vi "Mindsensors Numeric Pad Config.vi"(10 "Node Data":T1, 11 "NXT":T3) -> ()   [LabVIEW 2010]
uses:
  <vilib>/NXT/Subs/LVHSConnector.ctl
  Datatypes/Node.ctl
  UI Controls/PlugInControls/Pluginbackground.ctl
  <vilib>/NXT/Block Support/nxt.ctl
  <vilib>/NXT/Block Support/HWPage.SensorMode.ctl
  <vilib>/Utility/miscctls.llb/LVPointTypeDef.ctl
  <vilib>/NXT/Block Support/HWPage.SensorType.ctl
  ConvertNodeAddrSensor.vi
panel:
  in  "Node Data 2":T1
  out "error out":errorcluster
  out "NXTObject dup":T2 {"nxtIterHandle" format="%08x"; "modIterHandle" format="%08x"; "moduleHandle" format="%08x"; "fileIterHandle" format="%08x"; "fileHandle" format="%08x"; "nxtHandle" format="%08x"}
  in  "Numeric Pad":string
  out "Input Port":sgl
  out "Device Addr":u8 format="%x"
  out "number":i8
  out "#":bool
  out "9":bool
  out "6":bool
  out "3":bool
  out "0":bool
  out "8":bool
  out "5":bool
  out "2":bool
  out "*":bool
  out "7":bool
  out "4":bool
  out "1":bool
  out "?":dbl format="%#.2g"
  in  "Device Address":string
  in  "NXT Port":string
  in  "Name":string
  out "Headline":string="Type (auto populated)"
  in  "Sensor Parameters":string
  in  "Instance Specific Data":cluster{"Example Data":dbl}
  in  "Reset":bool
  in  "Save":bool
  in  "Stop":bool
  out "Background":T4=TRUE
  # "<- No controls below this line"
  # "Common controls such as Buttons, Rings, Sliders, Graphs, Decorations, etc can be found in the <labview>\\Targets\\NI\\NXT\\NXT Toolkit\\Schematic Editor\\UI Controls\\Plugin Controls\\ folder. Use these controls when possible to ensure a consistent look and feel with LabVIEW Education Edition."
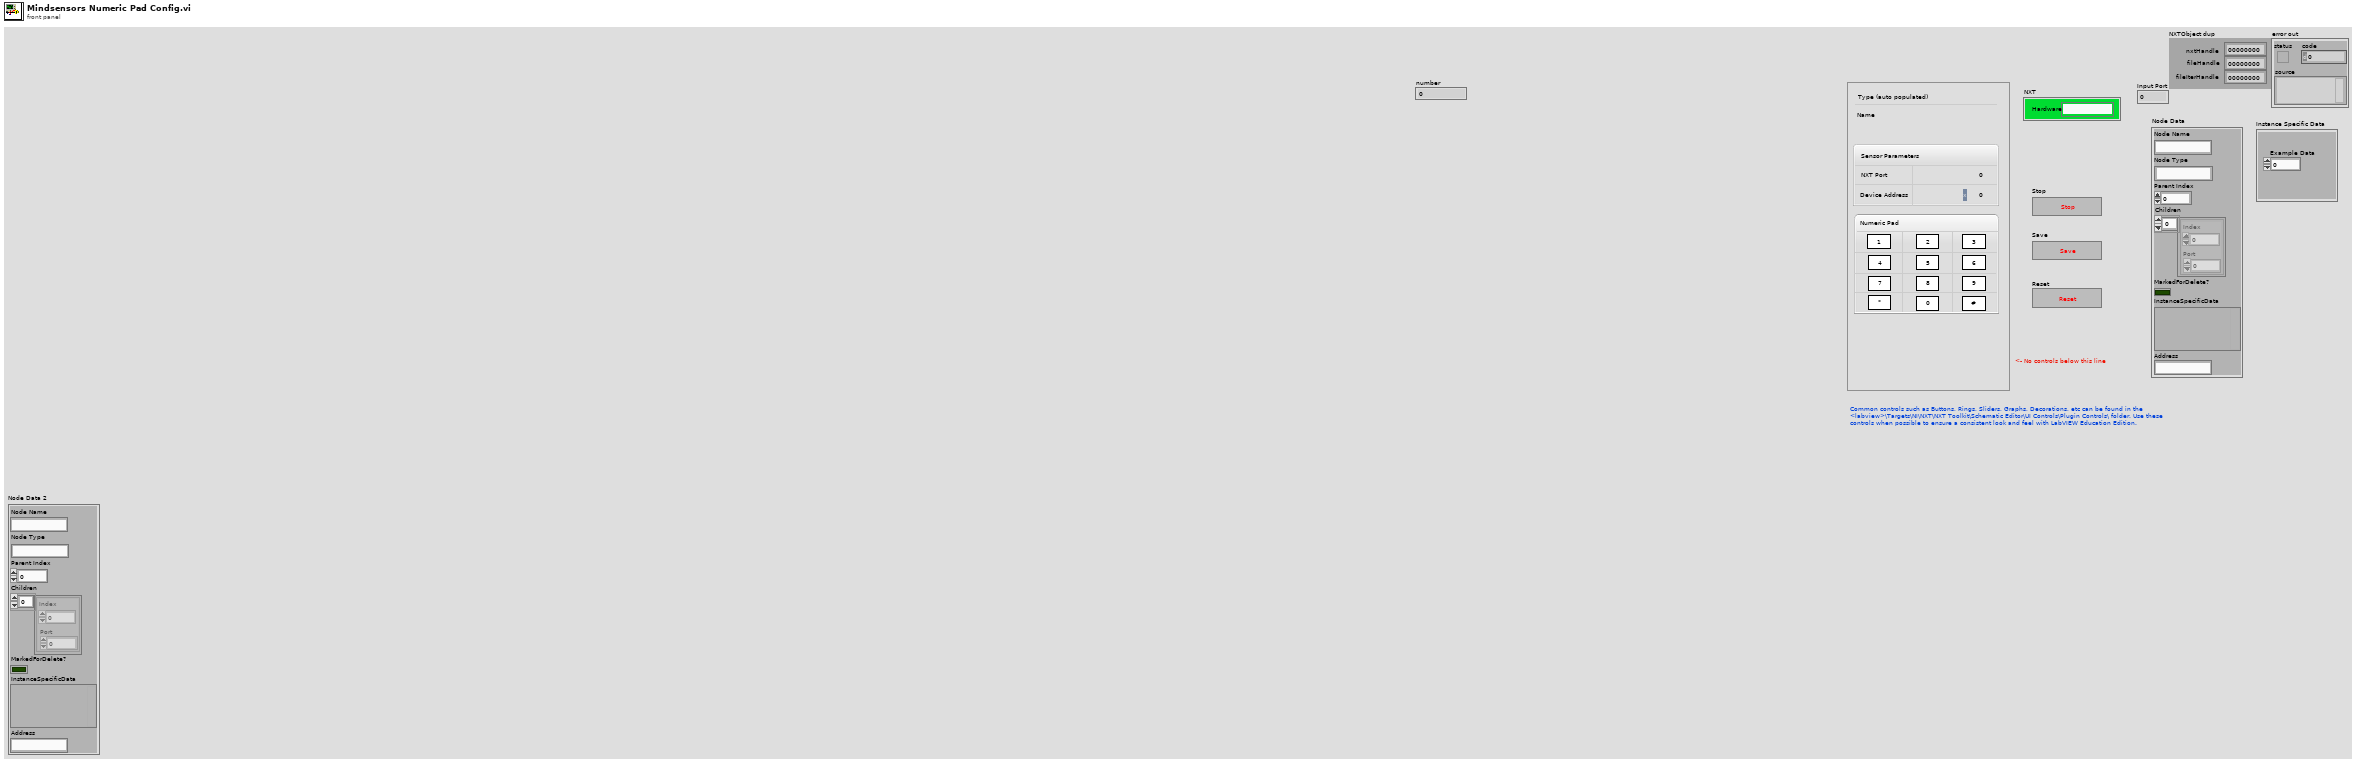
[diagram p1: front panel]
types:
  T1 = typedef "Node.ctl" = cluster{"Node Name":string, "Node Type":string, "Parent Index":i16, "Children":cluster{"Index":u16, "Port":u16}[], "MarkedForDelete?":bool, "InstanceSpecificData":variant, "Address":string}
  T2 = typedef "nxt.ctl" = cluster{"nxtHandle":u32, "fileHandle":u32, "fileIterHandle":u32, "moduleHandle":u32, "modIterHandle":u32, "nxtIterHandle":u32}
  T3 = typedef "LVHSConnector.ctl" = cluster{"Hardware":string, "Flattened String":string}
  T4 = typedef "Pluginbackground.ctl" = bool
  T5 = typedef "HWPage.SensorMode.ctl" = u8
  T6 = typedef "LVPointTypeDef.ctl" = cluster{"Horizontal":i16, "Vertical":i16}
  T7 = enum8{"Enabled", "Disabled", "Disabled and Grayed Out"}
  T8 = typedef "HWPage.SensorType.ctl" = u8
  T9 = typedef "NXT_InputPort.ctl" = u8
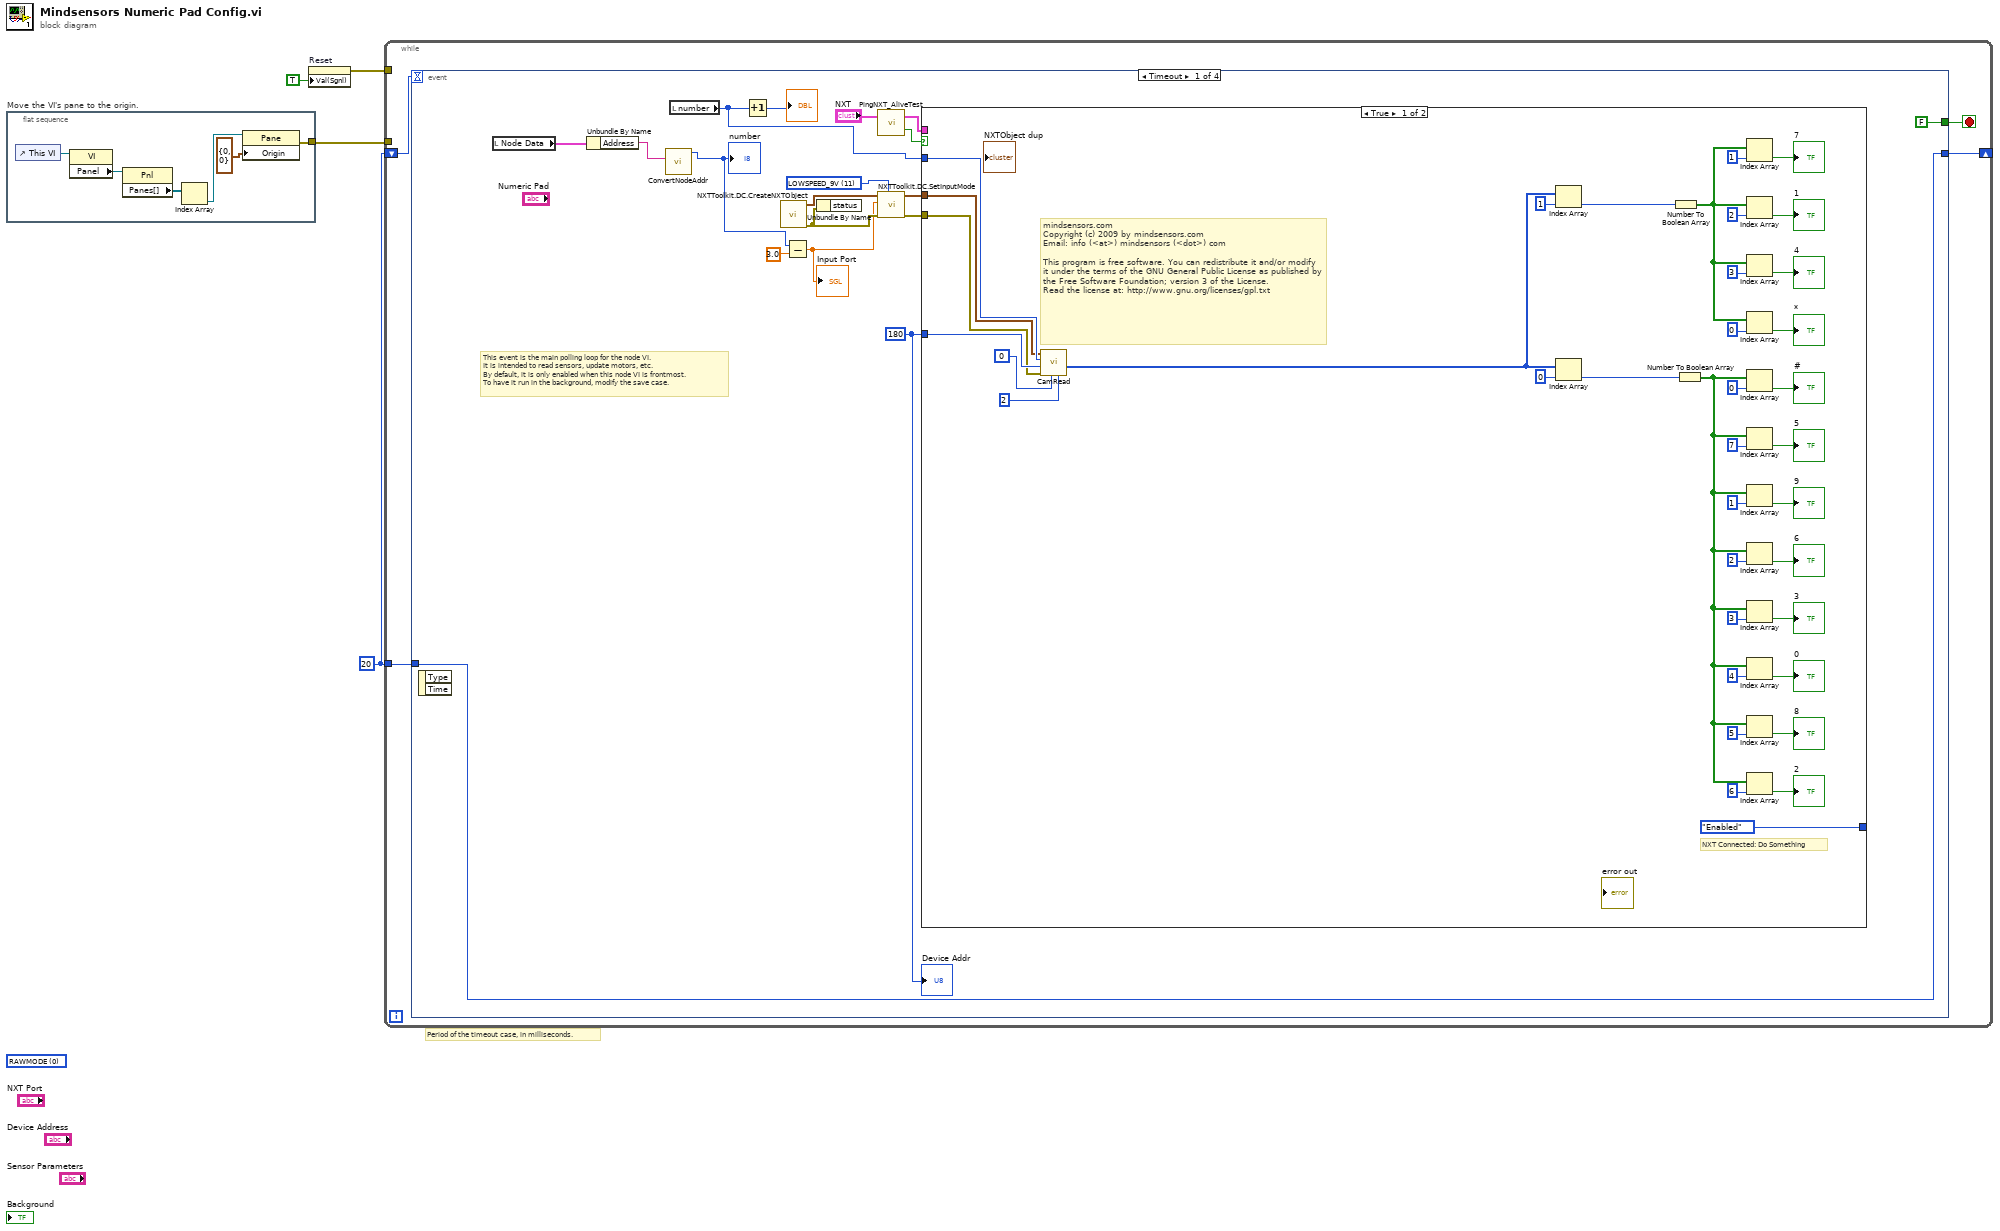
[diagram p0: block diagram]
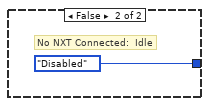
[diagram p2: hidden frame]
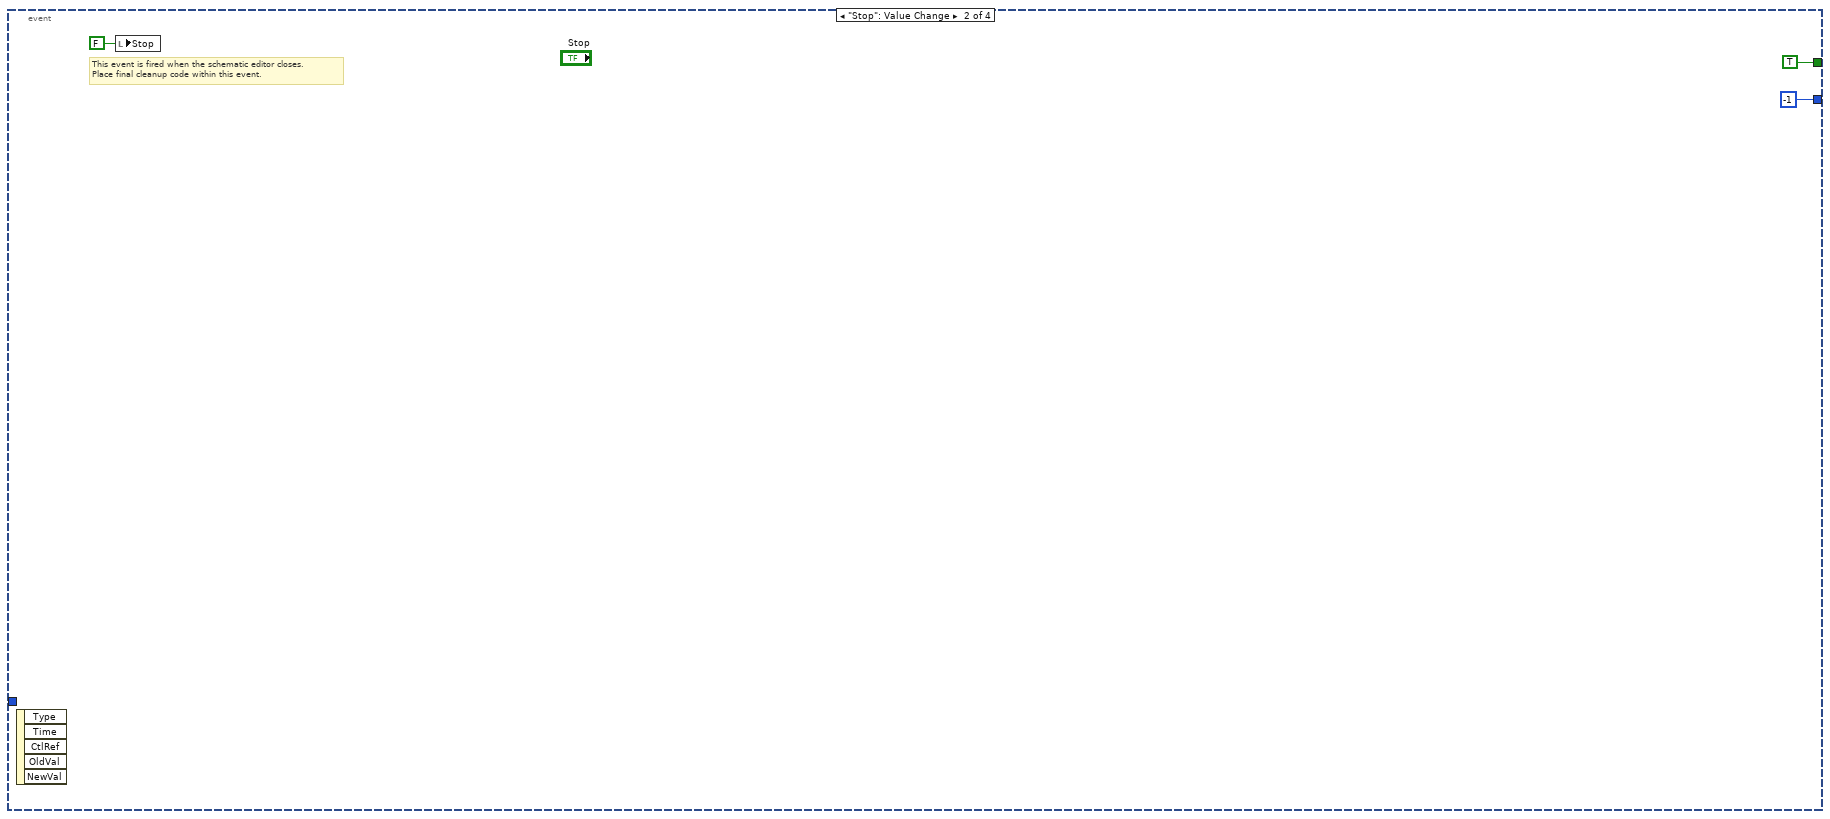
[diagram p3: hidden frame]
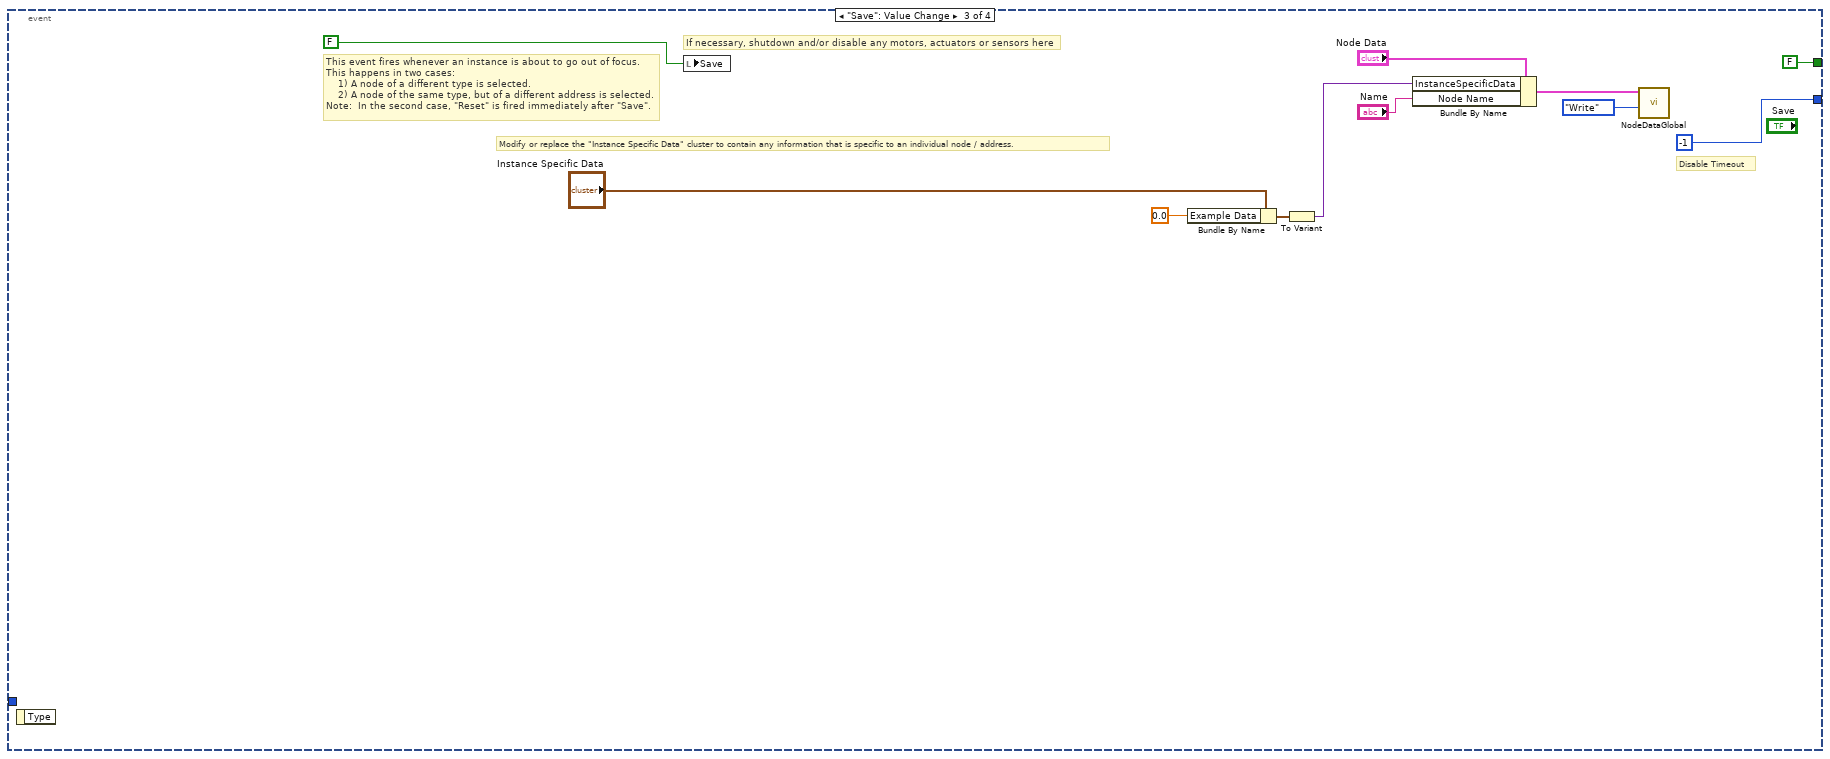
[diagram p4: hidden frame]
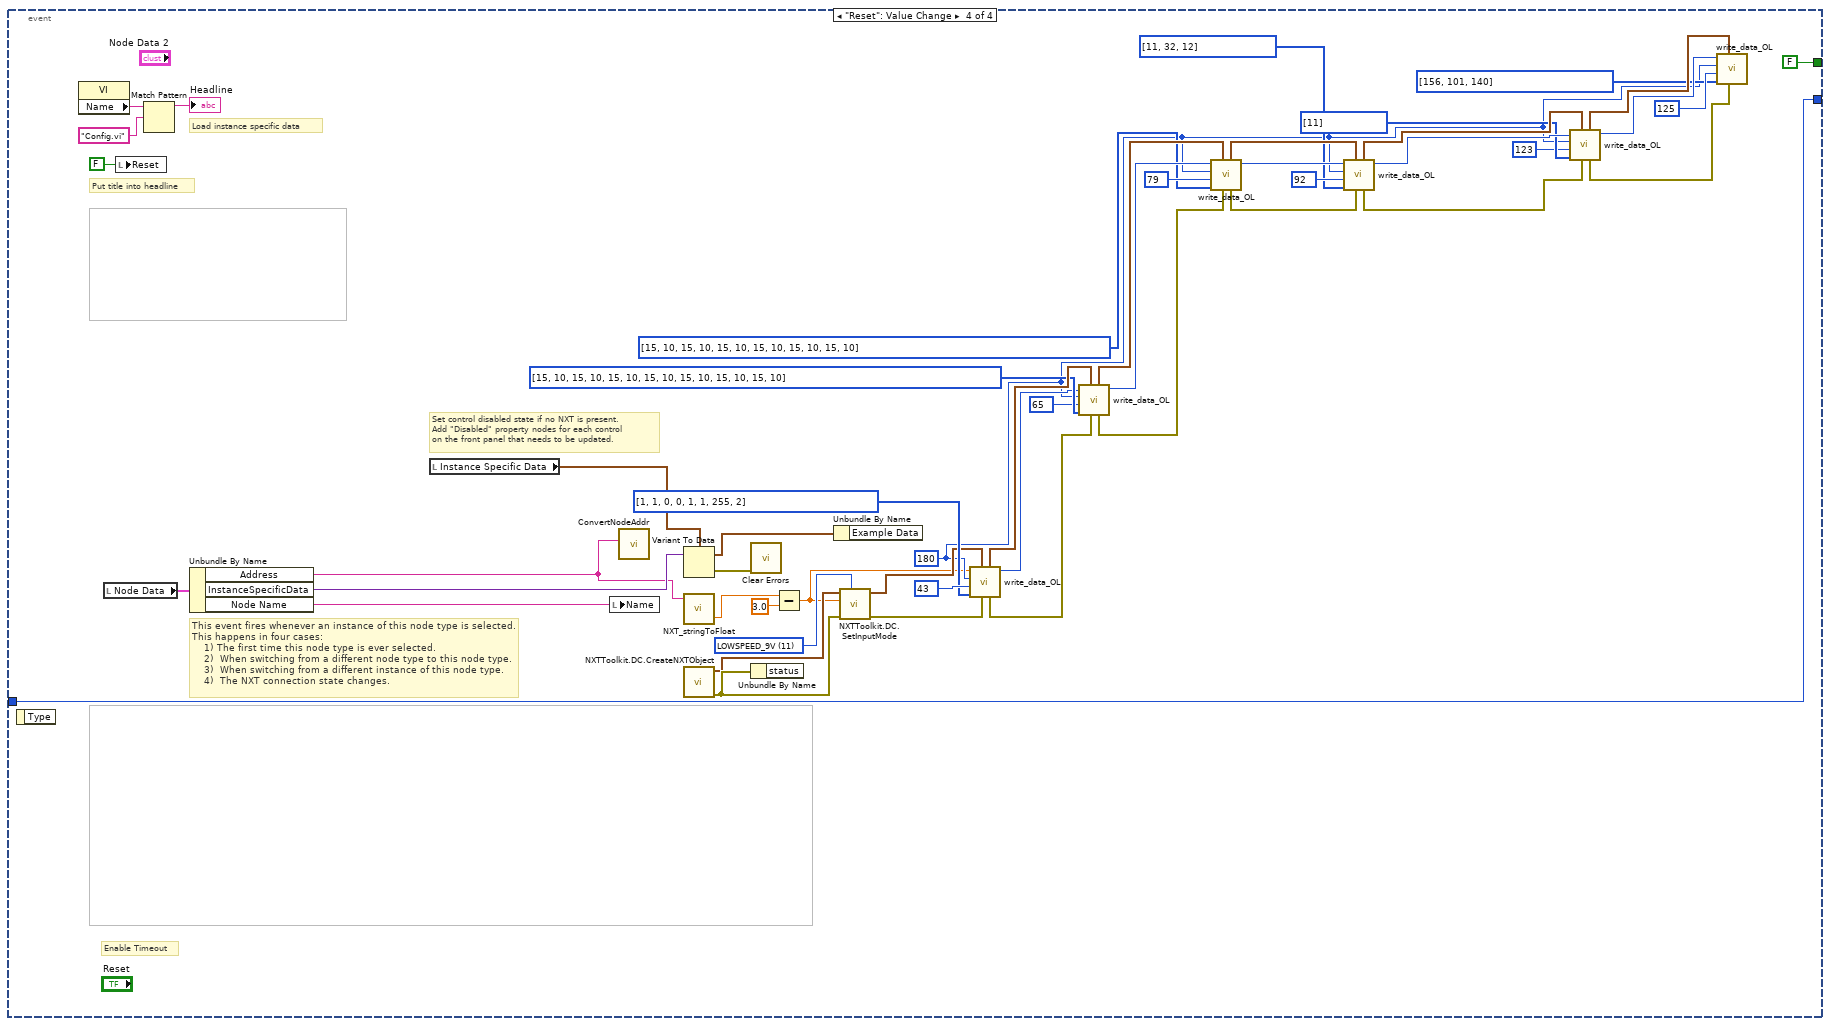
[diagram p5: hidden frame]
diagram:
  (unwired) T5 0 items=["RAWMODE"=0, "BOOLEANMODE"=32, "TRANSITIONCNTMODE"=64, "PERIODCOUNTERMODE"=96, "PCTFULLSCALEMODE"=128, "CELSIUSMODE"=160, "FAHRENHEITMODE"=192, "ANGLESTEPMODE"=224] ("Sensor Mode (RAWMODE)")
  w2 = 20
  # "Period of the timeout case, in milliseconds."
  n1 = flat-sequence "Move the VI's pane to the origin." {
    tunnel: [w5] -> w1
    frame #0 {
      n2 = control-ref of="This VI"() -> (w6:refnum<vi>)
      n3 = property class="VI"(reference=w6) -> ("Panel"=w7:refnum<vi>)  [unwired: 1 in, 2 out]
      n4 = property class="Pnl"(reference=w7) -> ("Panes[]"=w8:refnum<vi>[])  [unwired: 1 in, 2 out]
      n5 = Index Array(array=w8) -> (element=w9:refnum<vi>)  [unwired: 1 in]
      n6 = property class="Pane"(reference=w9, "Origin"=T6 {"Horizontal"=0, "Vertical"=0}) -> (error out=w5:errorcluster)  [unwired: 1 in, 1 out]
    }
  }
  n7 = property on="Reset" class="Bool (strict)"("Val(Sgnl)"=TRUE ("Value (Signaling)")) -> (error out=w3:errorcluster)  [unwired: 2 in, 1 out]
  n8 = while {
    tunnel: w3 -> [_]
    shift-right: [w12] -> _
    shift-left: w2 -> [w13]
    tunnel: w2 -> [w11]
    tunnel: w1 -> [_]
    stop <- w14 stop-if-true
    n9 = event shown="[0] Timeout" {
      selector: _ -> [_ _ _ _]
      dyn-events: _ -> [_ _ _ _]
      timeout: w13 -> [_ _ _ _]
      tunnel: [FALSE TRUE FALSE FALSE] -> w14
      tunnel: [w31 -1 -1 w130] -> w12
      tunnel: w11 -> [w31 _ _ w130]
      event Timeout {
        w24 = T8 11 items=["NO_SENSOR", "SWITCH", "TEMPERATURE", "REFLECTION", "ANGLE", "LIGHT_ACTIVE", "LIGHT_INACTIVE", "SOUND_DB", "SOUND_DBA", "CUSTOM", "LOWSPEED", "LOWSPEED_9V", "HIGHSPEED"] ("Sensor Type (NO_SENSOR)")
        w21 = 180 ("Registry Address")
        # "This event is the main polling loop for the node VI.\nIt is intended to read sensors, update motors, etc.\nBy default, it is only enabled when this node VI is frontmost.\nTo have it run in the background, modify the save case."
        n10 = event-data() -> ()  [unwired: 1 in, 2 out]
        n11 = local read "Node Data"() -> (w27:T1)
        n12 = Unbundle By Name(w27) -> ("Address"=w18:string)
        n13 = call-poly "ConvertNodeAddr.vi"("Sensor Port"=w18) -> ("NXT Port"=w17:T9)  [unwired: 6 in, 4 out]
        "number" <- w17
        n14 = local read "number"() -> (w15:i8)
        n15 = Increment(x=w15) -> (x+1=→"?":i8)
        n16 = call <vilib>:"NXTToolkit.DC.CreateNXTObject.vi"() -> ("error out"=w26:errorcluster, "NXTObject"=w25:T2)  [unwired: 9 in, 1 out]
        n17 = Subtract(x=w17, y=sgl 3.0) -> (x-y=w22:sgl)
        "Input Port" <- w22
        n18 = Unbundle By Name(w26) -> ()  [unwired: 1 out]
        n19 = call <vilib>:"PingNXT_AliveTest.vi"("NXT"="NXT") -> ("connected?"=w28:bool, "NXT"=w30:T3)  [unwired: 1 in]
        n20 = call <vilib>:"NXTToolkit.DC.SetInputMode.vi"("Sensor Type (NO_SENSOR)"=w24, "error in (no error)"=w26, "Input Port (Port 1)"=w22, "NXTObject"=w25) -> ("error out"=w19:errorcluster, "NXTObject dup"=w20:T2)  [unwired: 5 in, 1 out]
        n21 = case shown="True" w28 {
          tunnel: [T7."Enabled" ("Disabled") T7."Disabled" ("Disabled")] -> _
          tunnel: w30 -> [_ _]
          tunnel: w15 -> [w38 _]
          tunnel: w21 -> [w35 _]
          tunnel: w20 -> [w34 _]
          tunnel: w19 -> [w33 _]
          frame True {
            # "mindsensors.com\nCopyright (c) 2009 by mindsensors.com\nEmail: info (<at>) mindsensors (<dot>) com\n\nThis program is free software. You can redistribute it and/or modify\nit under the terms of the GNU General Public License as published by\nthe Free Software Foundation; version 3 of the License.\nRead the license at: http://www.gnu.org/licenses/gpl.txt"
            # "NXT Connected: Do Something"
            n22 = call <vilib>:"CamRead.vi"("bytes to read"=u8 2, "Reg Address"=u8 0, "error in (no error)"=w33, "Device Address"=w35, "Input Port in"=w38, "NXTObject"=w34) -> ("data Buffer"=w68:u8[])  [unwired: 5 out]
            n23 = Index Array(array=w68, index=1) -> (element=w40:u8)
            n24 = Index Array(array=w68, index=0) -> (element=w39:u8)
            n25 = Number To Boolean Array(number=w40) -> (Boolean array=w53:bool[])
            n26 = Number To Boolean Array(number=w39) -> (Boolean array=w66:bool[])
            n27 = Index Array(array=w53, index=1) -> (element=→"7":bool)
            n28 = Index Array(array=w53, index=2) -> (element=→"1":bool)
            n29 = Index Array(array=w53, index=3) -> (element=→"4":bool)
            n30 = Index Array(array=w53, index=0) -> (element=→"*":bool)
            n31 = Index Array(array=w66, index=0) -> (element=→"#":bool)
            n32 = Index Array(array=w66, index=7) -> (element=→"5":bool)
            n33 = Index Array(array=w66, index=1) -> (element=→"9":bool)
            n34 = Index Array(array=w66, index=2) -> (element=→"6":bool)
            n35 = Index Array(array=w66, index=3) -> (element=→"3":bool)
            n36 = Index Array(array=w66, index=4) -> (element=→"0":bool)
            n37 = Index Array(array=w66, index=5) -> (element=→"8":bool)
            n38 = Index Array(array=w66, index=6) -> (element=→"2":bool)
          }
          frame False {
            # "No NXT Connected:  Idle"
          }
        }
        "Device Addr" <- w21
      }
      event "Stop": Value Change {
        # "This event is fired when the schematic editor closes.\nPlace final cleanup code within this event."
        n39 = event-data() -> ()  [unwired: 1 in, 5 out]
        n40 = local write "Stop"(FALSE ("stop")) -> ()
      }
      event "Save": Value Change {
        # "If necessary, shutdown and/or disable any motors, actuators or sensors here"
        # "Modify or replace the \"Instance Specific Data\" cluster to contain any information that is specific to an individual node / address."
        # "Disable Timeout"
        # "This event fires whenever an instance is about to go out of focus.\nThis happens in two cases:\n    1) A node of a different type is selected.\n    2) A node of the same type, but of a different address is selected.\nNote:  In the second case, \"Reset\" is fired immediately after \"Save\"."
        n41 = event-data() -> ()  [unwired: 1 in, 1 out]
        n42 = local write "Save"(FALSE ("stop")) -> ()
        n43 = Bundle By Name(cluster="Instance Specific Data", "Example Data"=0.0) -> (w76:cluster{"Example Data":dbl})
        n44 = To Variant(anything=w76) -> (Variant=w83:variant)
        n45 = Bundle By Name(cluster="Node Data", "InstanceSpecificData"=w83, "Node Name"="Name") -> (w82:T1)
        n46 = call "NodeDataGlobal.vi"("Action"=enum16{"Read", "Write"}."Write", "Node Data In"=w82) -> ()  [unwired: 8 in, 2 out]
      }
      event "Reset": Value Change {
        w90 = 180 ("Registry Address")
        w93 = T8 11 items=["NO_SENSOR", "SWITCH", "TEMPERATURE", "REFLECTION", "ANGLE", "LIGHT_ACTIVE", "LIGHT_INACTIVE", "SOUND_DB", "SOUND_DBA", "CUSTOM", "LOWSPEED", "LOWSPEED_9V", "HIGHSPEED"] ("Sensor Type (NO_SENSOR)")
        # "Set control disabled state if no NXT is present.\nAdd \"Disabled\" property nodes for each control\non the front panel that needs to be updated."
        # "Load instance specific data"
        # "Enable Timeout"
        # "This event fires whenever an instance of this node type is selected.\nThis happens in four cases:\n    1) The first time this node type is ever selected.\n    2)  When switching from a different node type to this node type.\n    3)  When switching from a different instance of this node type. \n    4)  The NXT connection state changes."
        # "Put title into headline"
        n47 = event-data() -> ()  [unwired: 1 in, 1 out]
        n48 = property class="VI"() -> ("Name"=w126:string)  [unwired: 2 in, 2 out]
        n49 = local read "Node Data"() -> (w131:T1)
        n50 = local write "Reset"(FALSE ("Reset")) -> ()
        n51 = Match Pattern(string=w126, regular expression="Config.vi") -> (before substring=→"Headline":string)  [unwired: 1 in, 3 out]
        n52 = Unbundle By Name(w131) -> ("Address"=w89:string, "InstanceSpecificData"=w132:variant, "Node Name"=w124:string)
        n53 = local read "Instance Specific Data"() -> (w129:cluster{"Example Data":dbl})
        n54 = local write "Name"(w124) -> ()
        n55 = call-poly "ConvertNodeAddr.vi"("Sensor Port"=w89) -> ()  [unwired: 6 in, 5 out]
        n56 = Variant To Data(Variant=w132, type=w129) -> (error out=w128:errorcluster, data=w123:cluster{"Example Data":dbl})  [unwired: 1 in]
        n57 = call <vilib>:"NXT_stringToFloat.vi"("string"=w89) -> ("number"=w88:sgl)  [unwired: 2 in, 1 out]
        n58 = call <vilib>:"NXTToolkit.DC.CreateNXTObject.vi"() -> ("error out"=w95:errorcluster, "NXTObject"=w94:T2)  [unwired: 9 in, 1 out]
        n59 = call <vilib>:"Clear Errors.vi"("error in (no error)"=w128) -> ()  [unwired: 6 in, 1 out]
        n60 = Unbundle By Name(w95) -> ()  [unwired: 1 out]
        n61 = Subtract(x=w88, y=sgl 3.0) -> (x-y=w86:sgl)
        n62 = Unbundle By Name(w123) -> ()  [unwired: 1 out]
        n63 = call <vilib>:"NXTToolkit.DC.SetInputMode.vi"("Sensor Type (NO_SENSOR)"=w93, "error in (no error)"=w95, "Input Port (Port 1)"=w86, "NXTObject"=w94) -> ("error out"=w91:errorcluster, "NXTObject dup"=w92:T2)  [unwired: 5 in, 1 out]
        n64 = call <vilib>:"write_data_OL.vi"("error in (no error)"=w91, "NXTObject"=w92, "Data bytes"=u8[] [1, 1, 0, 0, 1, 1, 255, 2], "Reg Address"=u8 43, "Device Address"=w90, "Input Port in"=w86) -> ("Input Port dup"=w116:T9, "error out"=w114:errorcluster, "NXTObject dup"=w120:T2)  [unwired: 1 in, 2 out]
        n65 = call <vilib>:"write_data_OL.vi"("error in (no error)"=w114, "NXTObject"=w120, "Data bytes"=u8[] [15, 10, 15, 10, 15, 10, 15, 10, 15, 10, 15, 10, 15, 10], "Reg Address"=u8 65, "Device Address"=w90, "Input Port in"=w116) -> ("Input Port dup"=w115:T9, "error out"=w113:errorcluster, "NXTObject dup"=w117:T2)  [unwired: 1 in, 2 out]
        n66 = call <vilib>:"write_data_OL.vi"("error in (no error)"=w113, "NXTObject"=w117, "Data bytes"=u8[] [15, 10, 15, 10, 15, 10, 15, 10, 15, 10, 15, 10], "Reg Address"=u8 79, "Device Address"=w90, "Input Port in"=w115) -> ("Input Port dup"=w110:T9, "error out"=w106:errorcluster, "NXTObject dup"=w109:T2)  [unwired: 1 in, 2 out]
        n67 = call <vilib>:"write_data_OL.vi"("error in (no error)"=w106, "NXTObject"=w109, "Data bytes"=i32[] [11, 32, 12], "Reg Address"=u8 92, "Device Address"=w90, "Input Port in"=w110) -> ("Input Port dup"=w105:T9, "error out"=w103:errorcluster, "NXTObject dup"=w104:T2)  [unwired: 1 in, 2 out]
        n68 = call <vilib>:"write_data_OL.vi"("error in (no error)"=w103, "NXTObject"=w104, "Data bytes"=i32[] [11], "Reg Address"=u8 123, "Device Address"=w90, "Input Port in"=w105) -> ("Input Port dup"=w98:T9, "error out"=w99:errorcluster, "NXTObject dup"=w100:T2)  [unwired: 1 in, 2 out]
        n69 = call <vilib>:"write_data_OL.vi"("error in (no error)"=w99, "NXTObject"=w100, "Data bytes"=u8[] [156, 101, 140], "Reg Address"=u8 125, "Device Address"=w90, "Input Port in"=w98) -> ()  [unwired: 1 in, 5 out]
      }
    }
  }
